vi "put chess.vi"(1 "Chess Array":i32[][](array[numeric])=[[140, 130, 120, 110, 100, 111, 121, 131, 141], [-1, -1, -1, -1, -1, -1, -1, -1, -1], [-1, 150, -1, -1, -1, -1, -1, 151, -1], [160, -1, 161, -1, 162, -1, 163, -1, 164], [-1, -1, -1, -1, -1, -1, -1, -1, -1], [-1, -1, -1, -1, -1, -1, -1, -1, -1], [260, -1, 261, -1, 262, -1, 263, -1, 264], [-1, 250, -1, -1, -1, -1, -1, 251, -1], [-1, -1, -1, -1, -1, -1, -1, -1, -1], [240, 230, 220, 210, 200, 211, 221, 231, 241]], 2 "In Pic":picture) -> (0 "Out Pic":picture)   [LabVIEW 2009]
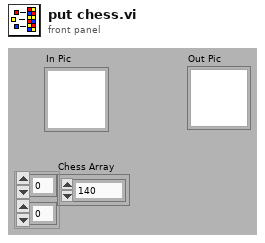
[diagram p1: front panel]
types:
  T1 = cluster{"Left":i32, "Top":i32, "Right":i32, "Bottom":i32}
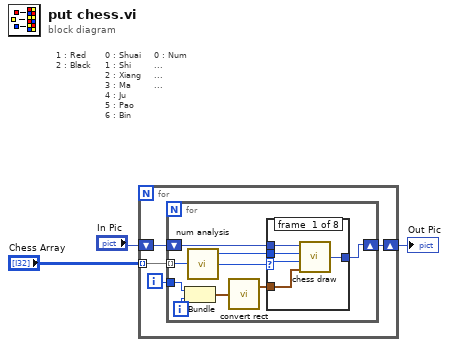
[diagram p0: block diagram]
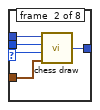
[diagram p2: hidden frame]
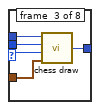
[diagram p3: hidden frame]
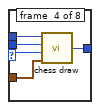
[diagram p4: hidden frame]
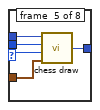
[diagram p5: hidden frame]
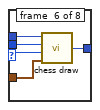
[diagram p6: hidden frame]
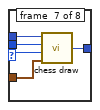
[diagram p7: hidden frame]
diagram:
  # "0 : Num\n...\n...\n..."
  # "0 : Shuai\n1 : Shi\n2 : Xiang\n3 : Ma\n4 : Ju\n5 : Pao\n6 : Bin"
  # "1 : Red\n2 : Black"
  n1 = for {
    tunnel: "Chess Array" -> [w7] mode=indexing
    shift-right: [w4] -> w1
    shift-left: "In Pic" -> [w5]
    i -> [w6]
    n2 = for {
      tunnel: w7 -> [w16] mode=indexing
      tunnel: w6 -> [w12]
      shift-right: [w8] -> w4
      shift-left: w5 -> [w9]
      i -> [w13]
      n3 = Bundle(w12, w13) -> (w14:cluster{i32, i32})  [unwired: 1 out]
      n4 = call "num analysis.vi"("x"=w16) -> ("Color"=w10:i32, "Chess"=w15:i32)  [unwired: 1 out]
      n5 = call "convert rect.vi"("Array Position"=w14) -> ("Output Rect"=w11:T1)  [unwired: 1 out]
      n6 = case shown="3" w15 {
        selector: w15 -> [w19 w24 w29 w34 w39 w44 w49 _]
        tunnel: w11 -> [w18 w23 w28 w33 w38 w43 w48 _]
        tunnel: w10 -> [w20 w25 w30 w35 w40 w45 w50 _]
        tunnel: w9 -> [w21 w26 w31 w36 w41 w46 w51 w52]
        tunnel: [w17 w22 w27 w32 w37 w42 w47 w52] -> w8
        frame #0 {
          n7 = call "chess draw.vi"("rect"=w18, "Chess"=w19, "Color"=w20, "In Pic"=w21) -> ("Out Pic"=w17:picture)
        }
        frame #1 {
          n8 = call "chess draw.vi"("rect"=w23, "Chess"=w24, "Color"=w25, "In Pic"=w26) -> ("Out Pic"=w22:picture)
        }
        frame #2 {
          n9 = call "chess draw.vi"("rect"=w28, "Chess"=w29, "Color"=w30, "In Pic"=w31) -> ("Out Pic"=w27:picture)
        }
        frame #3 {
          n10 = call "chess draw.vi"("rect"=w33, "Chess"=w34, "Color"=w35, "In Pic"=w36) -> ("Out Pic"=w32:picture)
        }
        frame #4 {
          n11 = call "chess draw.vi"("rect"=w38, "Chess"=w39, "Color"=w40, "In Pic"=w41) -> ("Out Pic"=w37:picture)
        }
        frame #5 {
          n12 = call "chess draw.vi"("rect"=w43, "Chess"=w44, "Color"=w45, "In Pic"=w46) -> ("Out Pic"=w42:picture)
        }
        frame #6 {
          n13 = call "chess draw.vi"("rect"=w48, "Chess"=w49, "Color"=w50, "In Pic"=w51) -> ("Out Pic"=w47:picture)
        }
        frame #7 {
        }
      }
    }
  }
  "Out Pic" <- w1
